vi "TIFF_Extract_Useful_Metadata.vi"(8 "error in (no error)":errorcluster, 10 "Array of Metadata IN":T1(array[cluster]), 11 "Tag IDs":dbl[](array[numeric])) -> (0 "error out":errorcluster, 2 "Description":string, 3 "Array of useful Meatadata OUT":T1(array[cluster]))   [LabVIEW 2025]
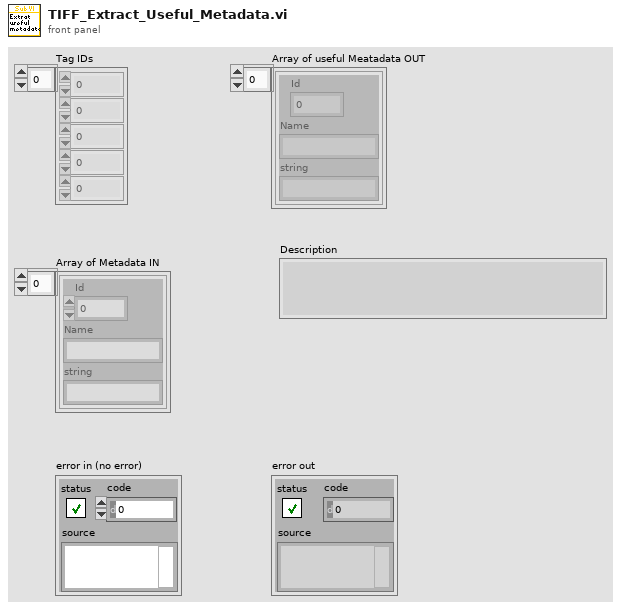
[diagram p1: front panel]
types:
  T1 = cluster{"Id":i32, "Name":string, "string":string}[]
  T2 = cluster{"Numeric":dbl, "Name":string, "string":string}
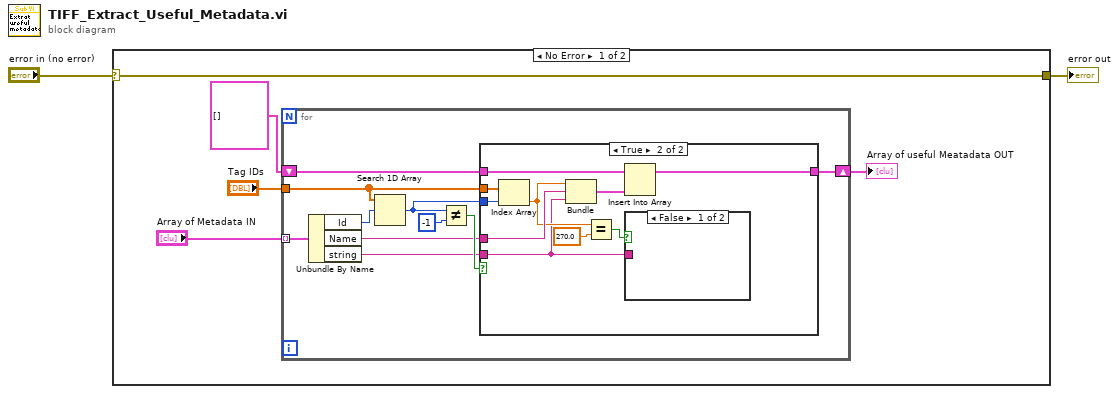
[diagram p0: block diagram]
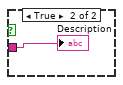
[diagram p3: hidden frame]
diagram:
  n1 = case shown="No Error" "error in (no error)" {
    selector: "error in (no error)" -> [w3 w30]
    tunnel: [w3 w30] -> w2
    frame No Error {
      n2 = for {
        tunnel: "Array of Metadata IN" -> [w12] mode=indexing
        shift-right: [w10] -> w6
        shift-left: T1 [] -> [w11]
        tunnel: "Tag IDs" -> [w8]
        n3 = Unbundle By Name(w12) -> ("Id"=w9:i32, "Name"=w14:string, "string"=w13:string)
        n4 = Search 1D Array(1D array=w8, element=w9) -> (index of element=w15:i32)  [unwired: 1 in]
        n5 = Not Equal?(x=w15, y=-1) -> (x != y?=w16:bool)
        n6 = case shown="True" w16 {
          tunnel: w15 -> [_ w23]
          tunnel: w14 -> [_ w28]
          tunnel: w13 -> [_ w19]
          tunnel: w11 -> [w18 w27]
          tunnel: [w18 w25] -> w10
          tunnel: w8 -> [_ w24]
          frame False {
          }
          frame True {
            n7 = Index Array(array=w24, index=w23) -> (element=w22:dbl)
            n8 = Bundle("Numeric"=w22, "Name"=w28, "string"=w19) -> (w26:T2)  [unwired: 1 in]
            n9 = Equal?(x=w22, y=270.0) -> (x = y?=w20:bool)
            n10 = Insert Into Array(array=w27, new element=w26) -> (w25:T1)  [unwired: 1 in]
            n11 = case shown="False" w20 {
              tunnel: w19 -> [_ w29]
              frame False {
              }
              frame True {
                "Description" <- w29
              }
            }
          }
        }
      }
      "Array of useful Meatadata OUT" <- w6
    }
    frame Error {
    }
  }
  "error out" <- w2
